vi "FTW-CodeGen-RelinkTerminals.vi"(0 "Diagram":refnum<vi>, 5 "Terms":T1(array[cluster]), 7 "PrototypeVI":refnum<vi>, 11 "error in":errorcluster) -> (4 "Diagram out":refnum<vi>, 15 "error out":errorcluster)   [LabVIEW 2014]
panel:
  # "Inputs"
  # "Outputs"
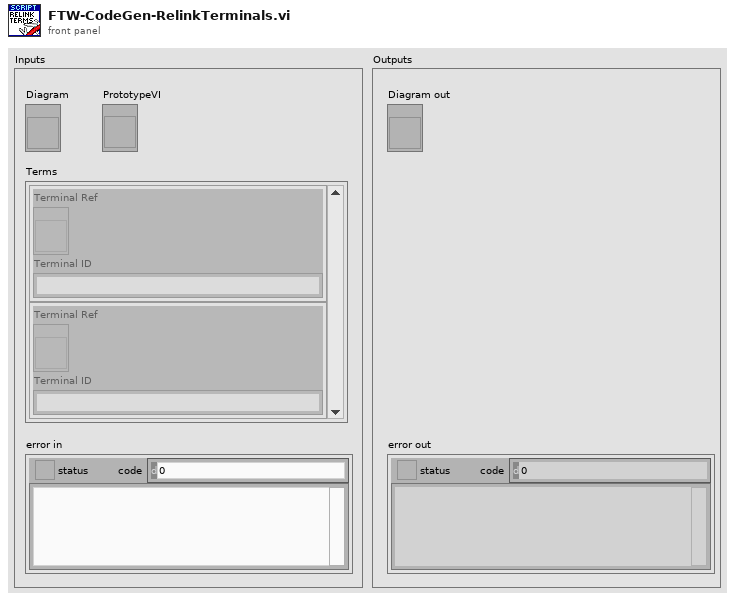
[diagram p1: front panel]
types:
  T1 = cluster{"Terminal Ref":refnum<vi>, "Terminal ID":string}[]
  T2 = typedef "LVPositionTypeDef.ctl" = cluster{"Left":i32, "Top":i32}
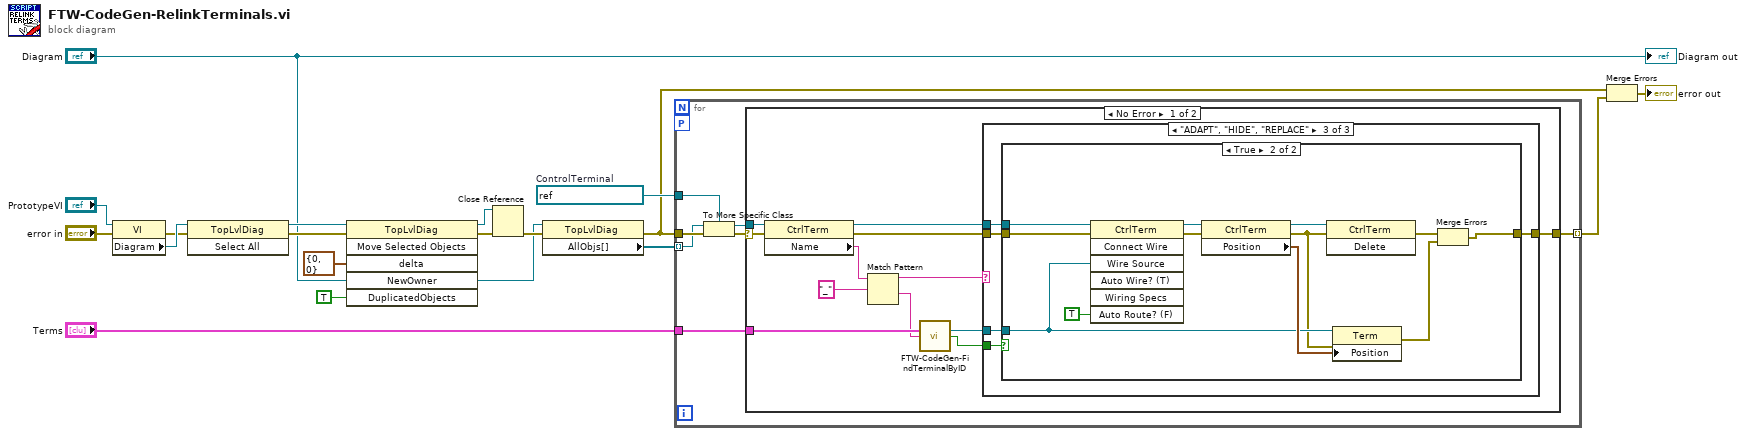
[diagram p0: block diagram]
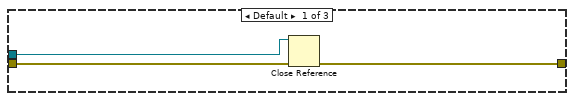
[diagram p2: hidden frame]
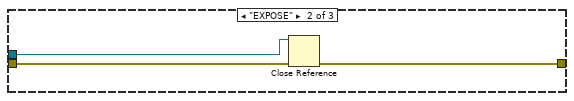
[diagram p3: hidden frame]
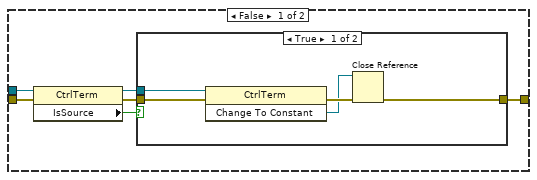
[diagram p4: hidden frame]
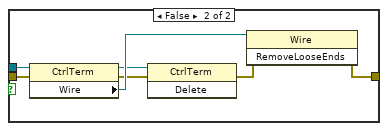
[diagram p5: hidden frame]
diagram:
  w16 = refnum<vi> refnum  # ControlTerminal
  n1 = property class="VI"(reference="PrototypeVI", error in="error in") -> (error out=w11:errorcluster, "Diagram"=w15:refnum<vi>)  [unwired: 1 out]
  n2 = invoke class="TopLvlDiag" method="Select All"(reference=w15, error in=w11) -> (reference out=w17:refnum<vi>, error out=w3:errorcluster)  [unwired: 1 in, 1 out]
  n3 = invoke class="TopLvlDiag" method="Move Selected Objects"(reference=w17, error in=w3, "delta"=cluster{"X":i32, "Y":i32} {"X"=0, "Y"=0} ("X/Y Delta"), "NewOwner"="Diagram", "DuplicatedObjects"=TRUE ("Duplicate? (F)")) -> (reference out=w10:refnum<vi>, error out=w9:errorcluster)  [unwired: 1 in, 4 out]
  n4 = Close Reference(reference=w10, error in (no error)=w9) -> (error out=w8:errorcluster)
  n5 = property class="TopLvlDiag"(reference="Diagram", error in=w8) -> (error out=w13:errorcluster, "AllObjs[]"=w4:refnum<vi>[])  [unwired: 1 out]
  n6 = for {
    tunnel: w4 -> [w19] mode=indexing
    tunnel: w13 -> [w20]
    tunnel: w16 -> [w25]
    tunnel: "Terms" -> [w22]
    tunnel: [w21] -> w14 mode=indexing
    workers-P: _ -> [_]
    n7 = To More Specific Class(target class=w25, reference=w19, error in=w20) -> (specific class reference=w23:refnum<vi>, error out=w24:errorcluster)
    n8 = case shown="No Error" w24 {
      selector: w24 -> [w36 _]
      tunnel: w23 -> [w37 _]
      tunnel: w22 -> [w31 _]
      tunnel: [w27 _] -> w21
      frame No Error {
        n9 = property class="CtrlTerm"(reference=w37, error in=w36) -> (reference out=w35:refnum<vi>, error out=w34:errorcluster, "Name"=w33:string)
        n10 = Match Pattern(string=w33, regular expression="_") -> (before substring=w26:string, after substring=w30:string)  [unwired: 1 in, 2 out]
        n11 = call "FTW-CodeGen-FindTerminalByID.vi"("Terms"=w31, "Terminal ID"=w30) -> ("Terminal Ref"=w28:refnum<vi>, "Found?"=w29:bool)  [unwired: 12 in]
        n12 = case shown="\"ADAPT\", \"HIDE\", \"REPLACE\"" w26 {
          tunnel: w35 -> [w39 w42 w48]
          tunnel: w34 -> [w40 w43 w47]
          tunnel: w29 -> [_ _ w46]
          tunnel: w28 -> [_ _ w45]
          tunnel: [w38 w41 w44] -> w27
          frame Default {
            n13 = Close Reference(reference=w39, error in (no error)=w40) -> (error out=w38:errorcluster)
          }
          frame "EXPOSE" {
            n14 = Close Reference(reference=w42, error in (no error)=w43) -> (error out=w41:errorcluster)
          }
          frame "ADAPT", "HIDE", "REPLACE" {
            n15 = case shown="True" w46 {
              tunnel: w45 -> [_ w68]
              tunnel: w48 -> [w49 w78]
              tunnel: w47 -> [w53 w77]
              tunnel: [w54 w69] -> w44
              frame False {
                n16 = property class="CtrlTerm"(reference=w49, error in=w53) -> (reference out=w52:refnum<vi>, error out=w50:errorcluster, "IsSource"=w51:bool)
                n17 = case shown="True" w51 {
                  tunnel: [w55 w64] -> w54
                  tunnel: w52 -> [w58 w66]
                  tunnel: w50 -> [w59 w65]
                  frame True {
                    n18 = invoke class="CtrlTerm" method="Change To Constant"(reference=w58, error in=w59) -> (error out=w57:errorcluster, "Change To Constant"=w56:refnum<vi>)  [unwired: 1 in, 1 out]
                    n19 = Close Reference(reference=w56, error in (no error)=w57) -> (error out=w55:errorcluster)
                  }
                  frame False {
                    n20 = property class="CtrlTerm"(reference=w66, error in=w65) -> (reference out=w62:refnum<vi>, error out=w61:errorcluster, "Wire"=w63:refnum<vi>)
                    n21 = invoke class="CtrlTerm" method="Delete"(reference=w62, error in=w61) -> (error out=w60:errorcluster)  [unwired: 1 in, 2 out]
                    n22 = invoke class="Wire" method="RemoveLooseEnds"(reference=w63, error in=w60) -> (error out=w64:errorcluster)  [unwired: 1 in, 2 out]
                  }
                }
              }
              frame True {
                n23 = invoke class="CtrlTerm" method="Connect Wire"(reference=w78, error in=w77, "Wire Source"=w68, "Auto Route? (F)"=TRUE) -> (reference out=w76:refnum<vi>, error out=w75:errorcluster)  [unwired: 3 in, 5 out]
                n24 = property class="CtrlTerm"(reference=w76, error in=w75) -> (reference out=w72:refnum<vi>, error out=w67:errorcluster, "Position"=w73:T2)
                n25 = invoke class="CtrlTerm" method="Delete"(reference=w72, error in=w67) -> (error out=w71:errorcluster)  [unwired: 1 in, 2 out]
                n26 = property class="Term"(reference=w68, error in=w67, "Position"=w73) -> (error out=w70:errorcluster)  [unwired: 1 out]
                n27 = Merge Errors(w71, w70) -> (w69:errorcluster)
              }
            }
          }
        }
      }
      frame Error {
      }
    }
  }
  n28 = Merge Errors(w13, w14) -> (→"error out":errorcluster)
  "Diagram out" <- "Diagram"
